vi "function2.vi"   [LabVIEW 2016, in "Test.lvrbt"]
uses:
  Test.lvrbt
  <vilib>/NXT/Subs/ColorSensorColors.ctl
  <vilib>/NXT/Block Support/NXT_InputPort.ctl
  <vilib>/NXT/Hardware/Plugins/Tetrix DC Motor/TetrixDCMotorAddress.ctl
  <vilib>/NXT/NXTIO Xnodes/NXTIONodeSubVIs/TETRIX IO Move DC Motors.vi
  <vilib>/NXT/Dual Mode Library/Waits/Wait_Num.vi
  <vilib>/NXT/NXTIO Xnodes/NXTIONodeSubVIs/TETRIX IO Stop DC Motors.vi
  <vilib>/NXT/Dual Mode Library/Waits/Wait_EV3_Color_Color.vi
  <vilib>/NXT/Subs/LVHSConnector.ctl
  <vilib>/NXT/NXTIO Xnodes/AddressXNode/NXTIOAddress.xnode
  <vilib>/NXT/NXTIO Xnodes/NXTIOXNode/NXTIO.xnode
  <vilib>/NXT/LegoClasses/BrickReference/BrickReference.lvclass
types:
  T1 = typedef "NXT_InputPort.ctl" = u32
  T2 = typedef "ColorSensorColors.ctl" = enum16{"No Color", "Black", "Blue", "Green", "Yellow", "Red", "White", "Brown"}
  T3 = typedef "TetrixDCMotorAddress.ctl" = i32
  T4 = typedef "LVHSConnector.ctl" = refnum<class "BrickReference.lvclass">
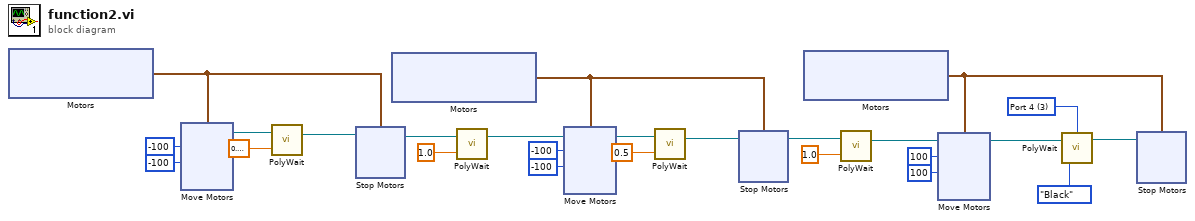
[diagram p0: block diagram]
diagram:
  w1 = T1 3 items=["Port 1", "Port 2", "Port 3", "Port 4"] ("Port (Port 1)")
  n1 = xnode "Motors"() -> ("Motor"=w21:cluster{"TetrixDCMotor":T3, "TetrixDCMotor":T3})
  n2 = xnode "Move Motors"("Power/Speed 2"=i8 -100, "Power/Speed 1"=i8 -100, "Motors"=w21) -> ("NXT/EV3"=w23:T4)  [unwired: 1 in]
  n3 = call-poly <vilib>:"PolyWait.vi"("Time (1 sec)"=sgl 0.6, "NXT/EV3"=w23) -> ("NXT/EV3"=w20:T4)  [unwired: 2 in]
  n4 = xnode "Stop Motors"("Motors"=w21, "NXT/EV3"=w20) -> ("NXT/EV3"=w12:T4)
  n5 = xnode "Motors"() -> ("Motor"=w15:cluster{"TetrixDCMotor":T3, "TetrixDCMotor":T3})
  n6 = call-poly <vilib>:"PolyWait.vi"("Time (1 sec)"=sgl 1.0, "NXT/EV3"=w12) -> ("NXT/EV3"=w11:T4)  [unwired: 2 in]
  n7 = xnode "Move Motors"("Power/Speed 2"=i8 -100, "Power/Speed 1"=i8 -100, "Motors"=w15, "NXT/EV3"=w11) -> ("NXT/EV3"=w17:T4)
  n8 = call-poly <vilib>:"PolyWait.vi"("Time (1 sec)"=sgl 0.5, "NXT/EV3"=w17) -> ("NXT/EV3"=w14:T4)  [unwired: 2 in]
  n9 = xnode "Stop Motors"("Motors"=w15, "NXT/EV3"=w14) -> ("NXT/EV3"=w9:T4)
  n10 = xnode "Motors"() -> ("Motor"=w2:cluster{"TetrixDCMotor":T3, "TetrixDCMotor":T3})
  n11 = call-poly <vilib>:"PolyWait.vi"("Time (1 sec)"=sgl 1.0, "NXT/EV3"=w9) -> ("NXT/EV3"=w8:T4)  [unwired: 2 in]
  n12 = xnode "Move Motors"("Power/Speed 2"=i8 100, "Power/Speed 1"=i8 100, "Motors"=w2, "NXT/EV3"=w8) -> ("NXT/EV3"=w5:T4)
  n13 = call-poly <vilib>:"PolyWait.vi"("Color (Red)"=ColorSensorColors."Black", "NXT/EV3"=w5, "Port (Port 1)"=w1) -> ("NXT/EV3"=w3:T4)  [unwired: 1 in]
  n14 = xnode "Stop Motors"("Motors"=w2, "NXT/EV3"=w3) -> ()  [unwired: 1 out]
